vi "Main.vi"() -> ()   [LabVIEW 2023]
uses:
  #type_def_Cafe_Additions.ctl
  #type_def_States.ctl
  #type_def_Coffee_Data.ctl
  #type_def_Timing.ctl
  <vilib>/Utility/file.llb/Write Delimited Spreadsheet (string).vi
panel:
  out "error out":errorcluster
  in  "error in":errorcluster
  in  "Stop":bool
  out "Cafe Additions":T1
  in  "Cafe Mocha":bool
  in  "Cafe Latte":bool
  in  "Espresso Macchiato":bool
  in  "Espresso":bool
  # "WYBIERZ KAWÊ:"
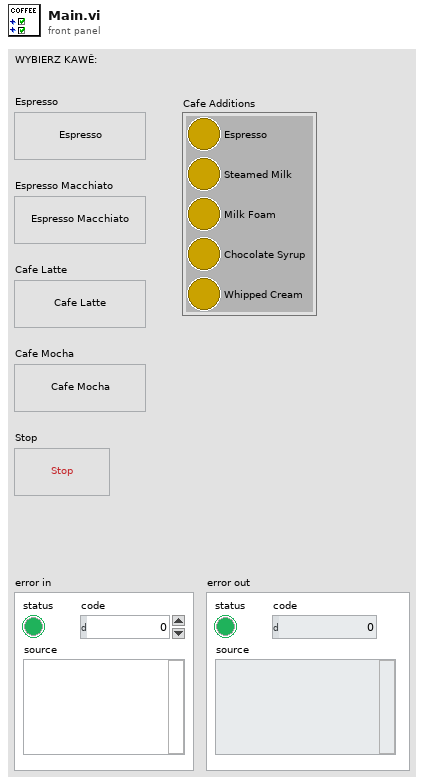
[diagram p1: front panel]
types:
  T1 = typedef "#type_def_Cafe_Additions.ctl" = cluster{"Espresso":bool, "Steamed Milk":bool, "Milk Foam":bool, "Chocolate Syrup":bool, "Whipped Cream":bool}
  T2 = typedef "#type_def_States.ctl" = enum16{"Init", "Idle", "Espresso", "Steamed Milk", "Milk Foam", "Chocolate Syrup", "Whipped Cream", "Stop", "Log"}
  T3 = typedef "#type_def_Coffee_Data.ctl" = cluster{"Cafe Additions":T1, "Timing":T4}
  T4 = typedef "#type_def_Timing.ctl" = cluster{"Espresso":dbl, "Steamed Milk":dbl, "Milk Foam":dbl, "Chocolate Syrup":dbl, "Whipped Cream":dbl}
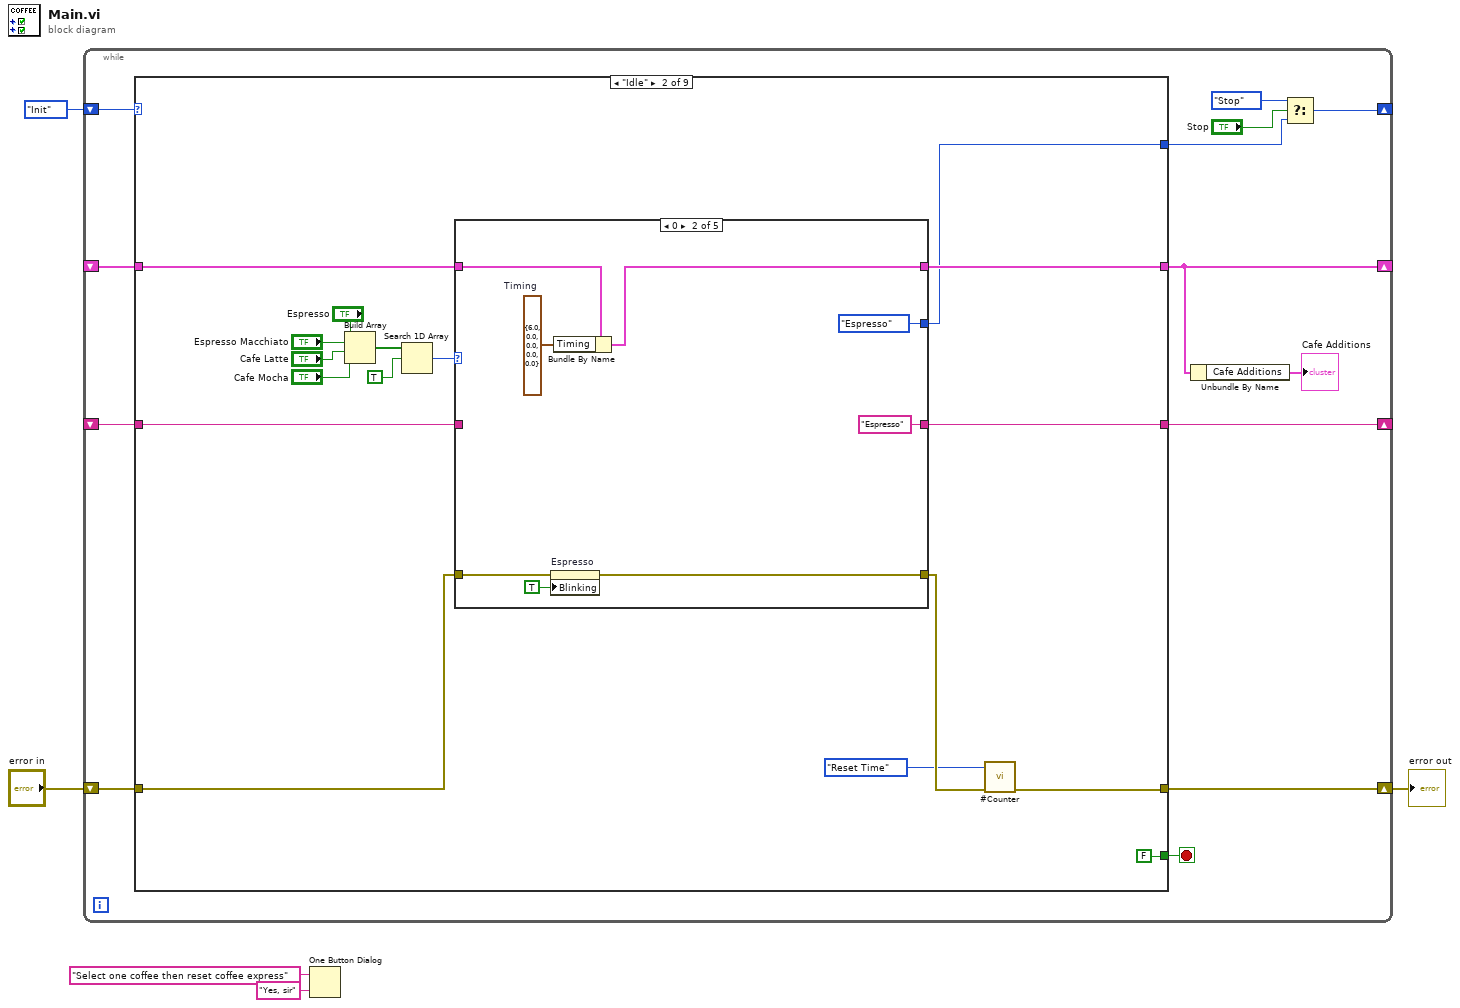
[diagram p0: block diagram]
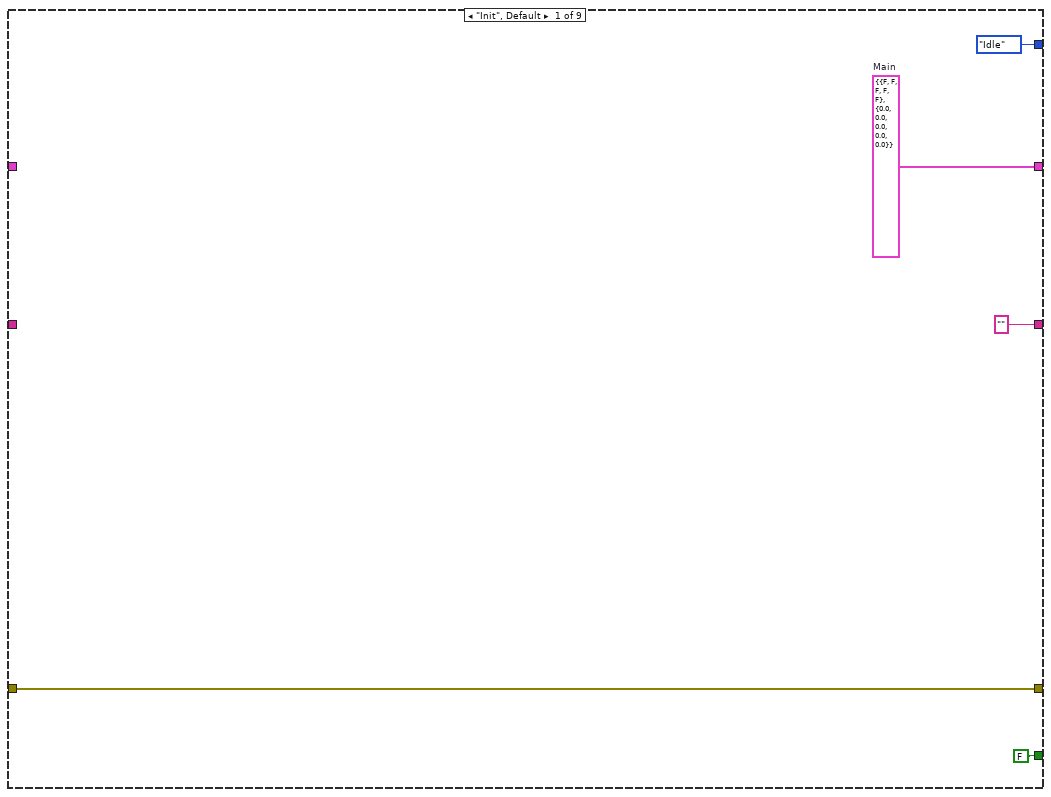
[diagram p2: hidden frame]
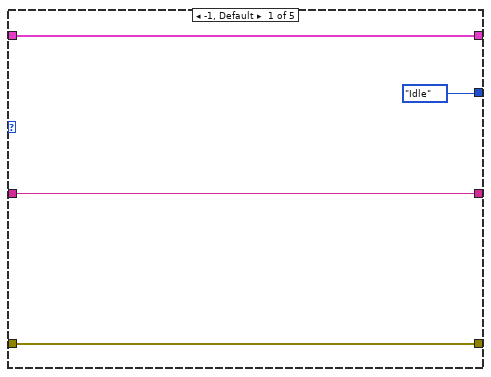
[diagram p3: hidden frame]
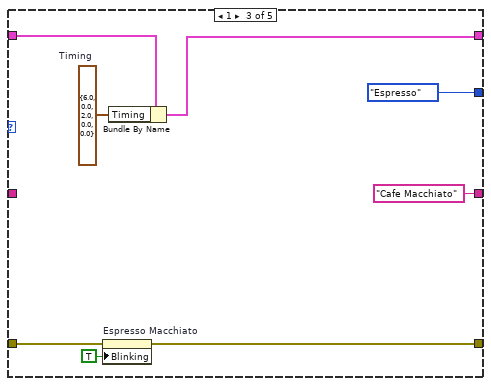
[diagram p4: hidden frame]
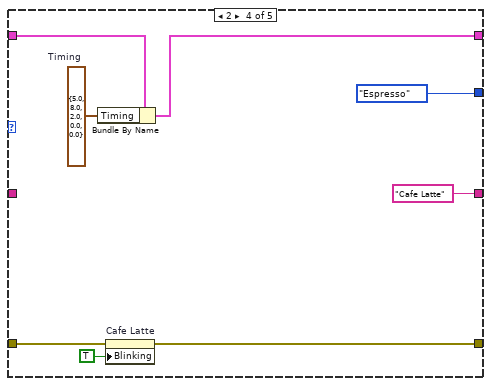
[diagram p5: hidden frame]
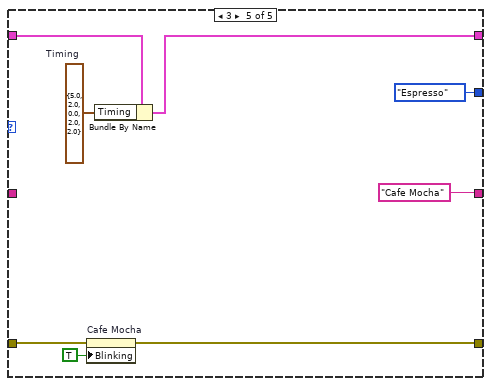
[diagram p6: hidden frame]
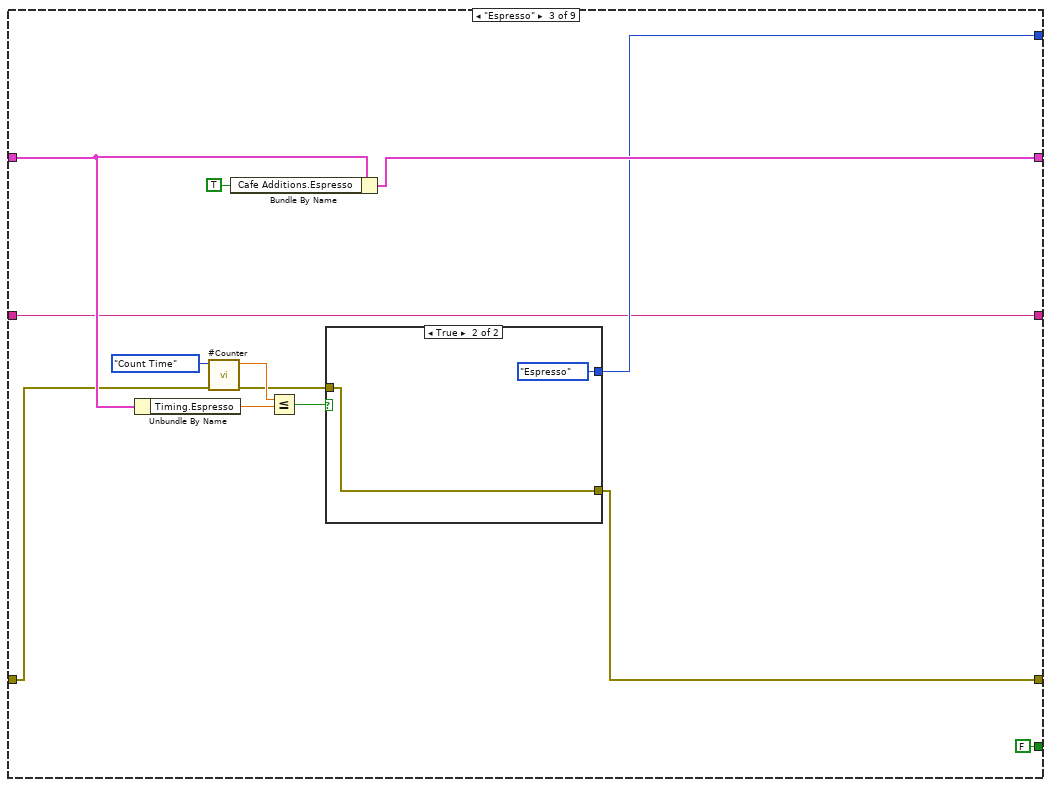
[diagram p7: hidden frame]
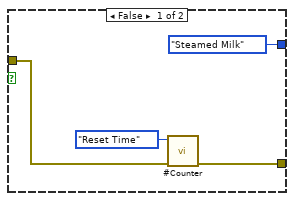
[diagram p8: hidden frame]
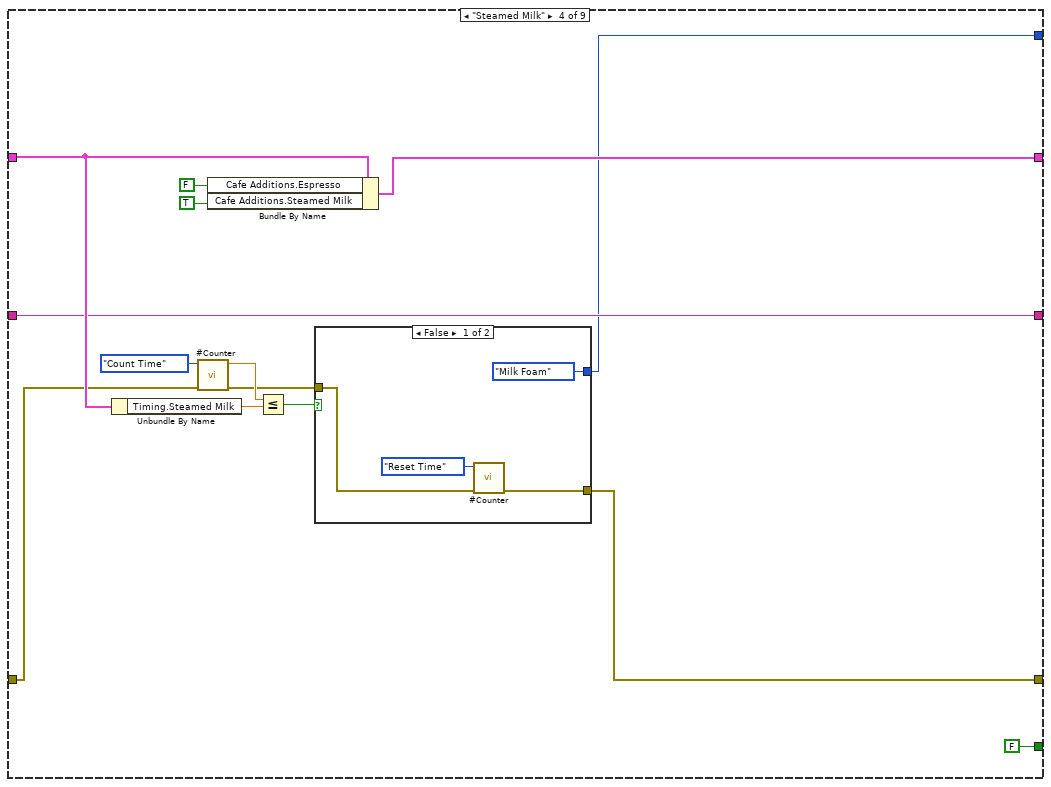
[diagram p9: hidden frame]
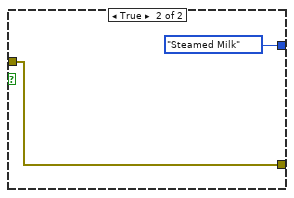
[diagram p10: hidden frame]
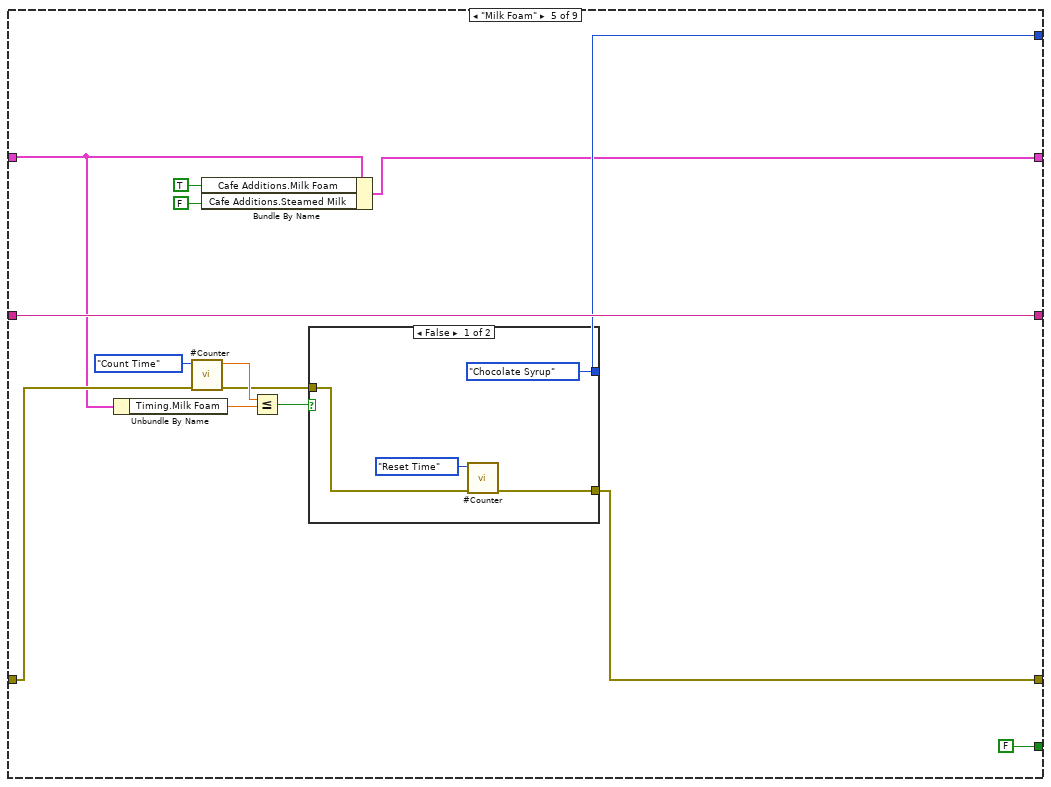
[diagram p11: hidden frame]
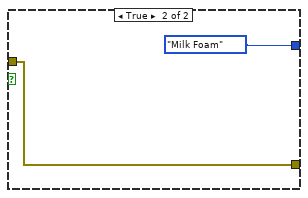
[diagram p12: hidden frame]
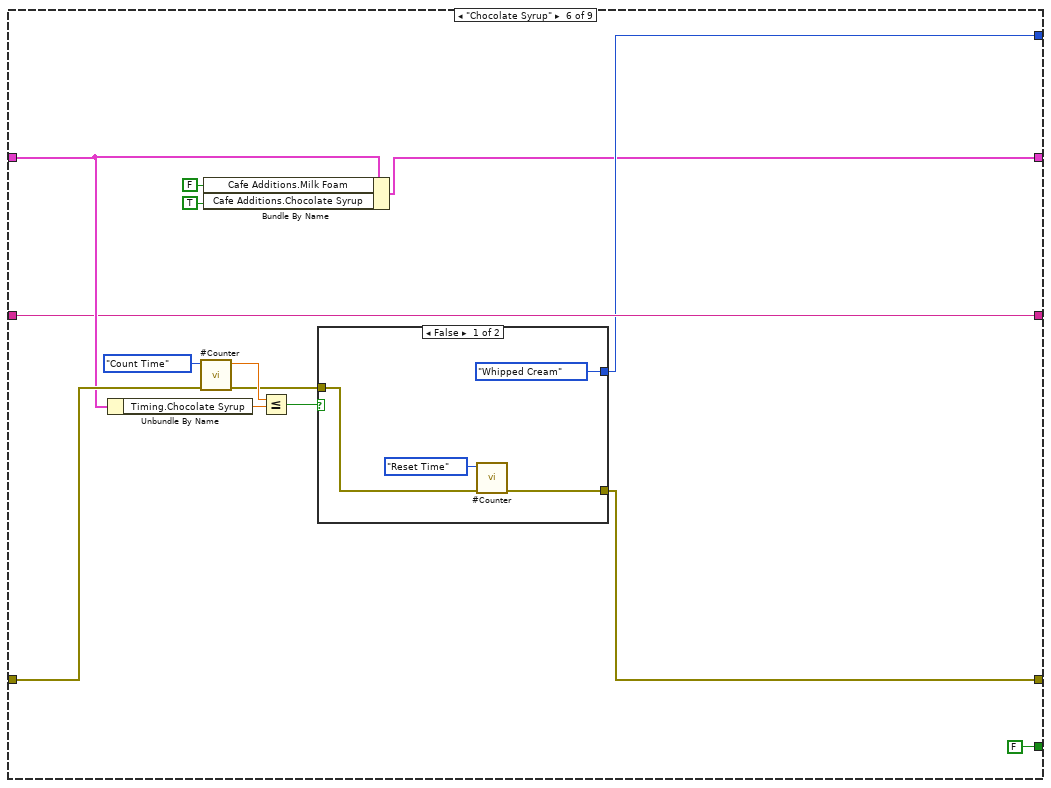
[diagram p13: hidden frame]
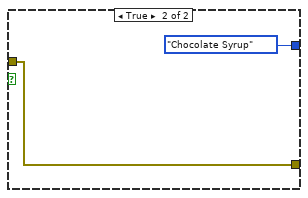
[diagram p14: hidden frame]
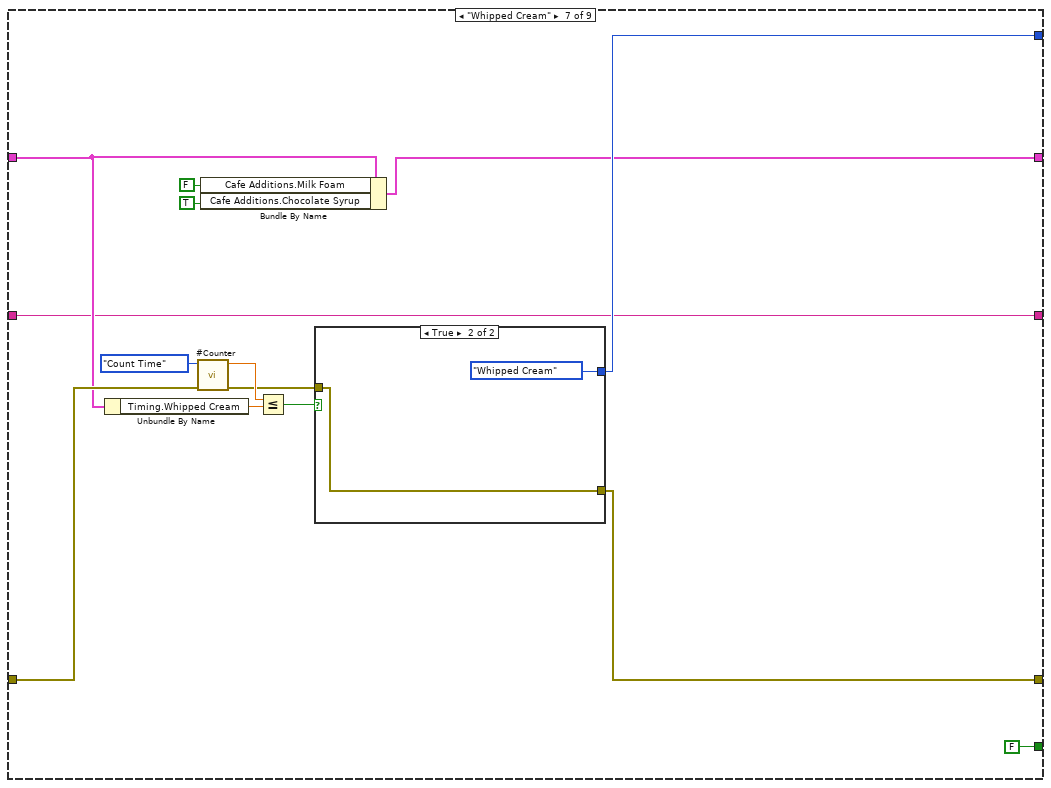
[diagram p15: hidden frame]
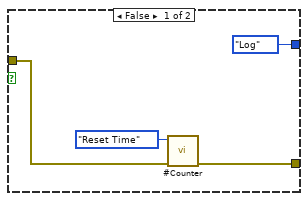
[diagram p16: hidden frame]
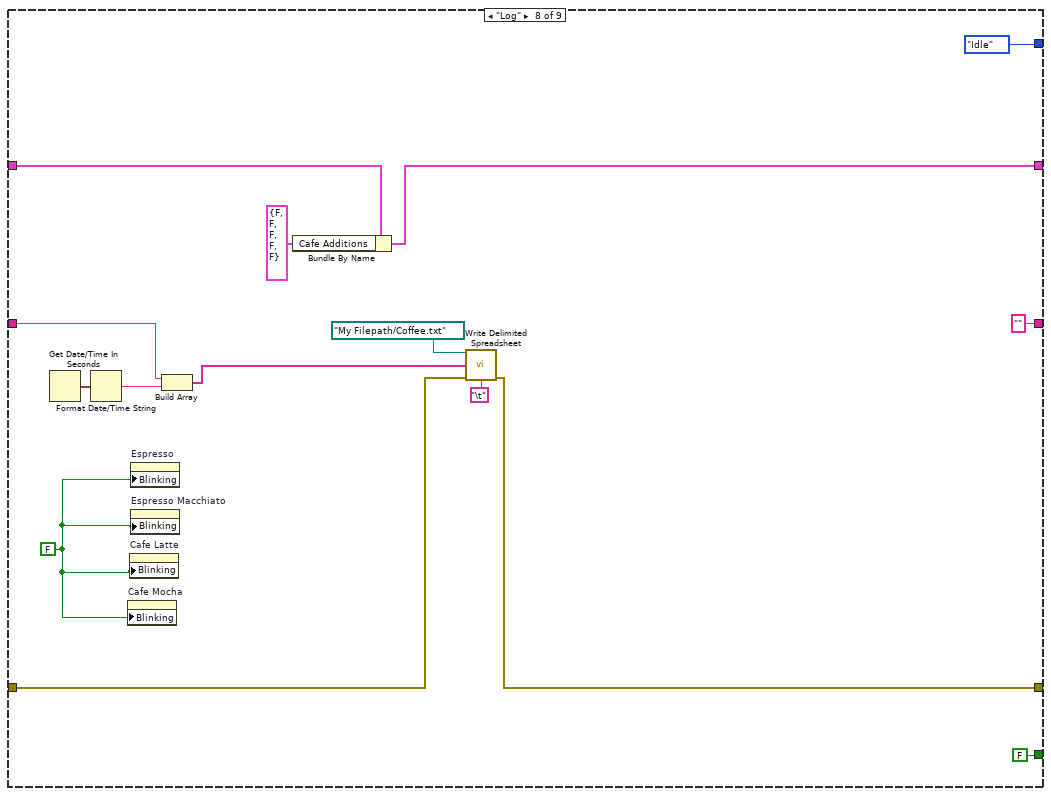
[diagram p17: hidden frame]
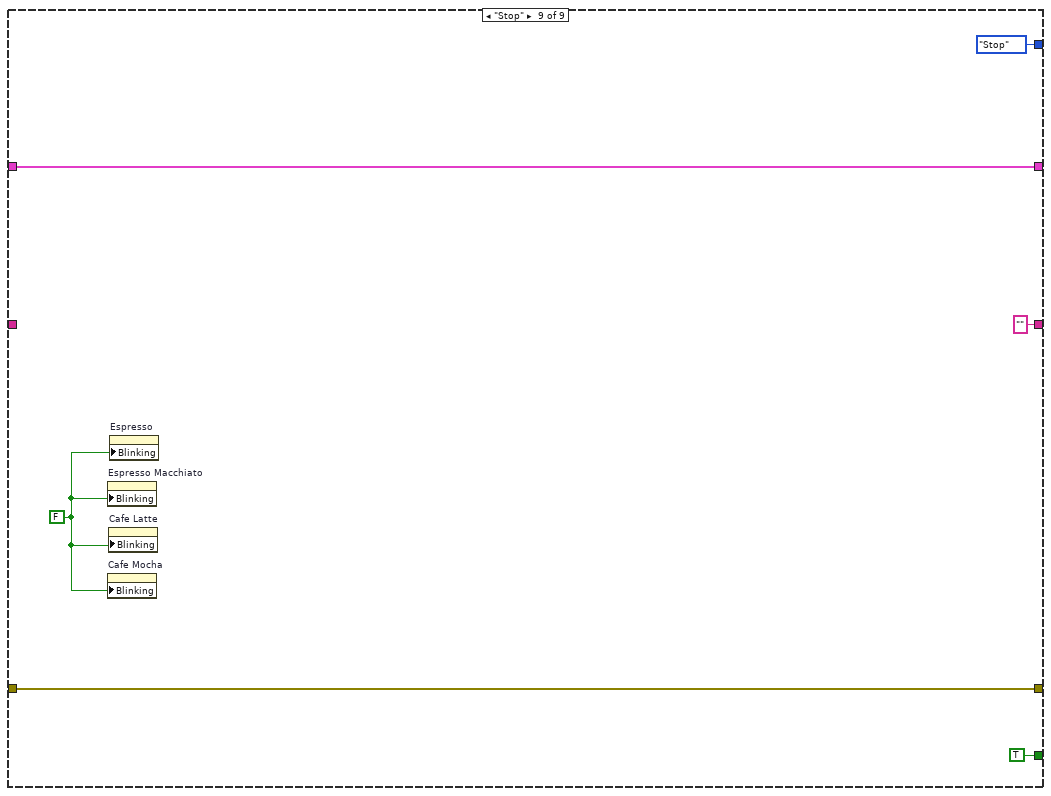
[diagram p18: hidden frame]
diagram:
  n1 = while {
    shift-right: [w17] -> w4
    shift-left: "error in" -> [w18]
    shift-right: [w6] -> _
    shift-left: #type_def_States."Init" -> [w16]
    shift-right: [w15] -> _
    shift-left: _ -> [w12]
    shift-right: [w13] -> _
    shift-left: _ -> [w11]
    stop <- w10 stop-if-true
    n2 = case shown="\"Idle\"" w16 {
      tunnel: w18 -> [w21 w37 w82 w102 w122 w141 w161 w189 w195]
      tunnel: [w21 w26 w80 w97 w119 w136 w159 w188 w195] -> w17
      tunnel: [w23 w33 w88 w100 w116 w137 w157 w183 w194] -> w15
      tunnel: ["" w35 w78 w101 w123 w139 w156 "" ""] -> w13
      tunnel: w12 -> [_ w34 w87 w103 w121 w140 w160 w184 w194]
      tunnel: w11 -> [_ w36 w78 w101 w123 w139 w156 w180 _]
      tunnel: [FALSE FALSE FALSE FALSE FALSE FALSE FALSE FALSE TRUE] -> w10
      tunnel: [#type_def_States."Idle" w32 w84 w96 w117 w138 w158 #type_def_States."Idle" #type_def_States."Stop"] -> w7
      frame "Init", Default {
        w23 = T3 {"Cafe Additions"={"Espresso"=FALSE, "Steamed Milk"=FALSE, "Milk Foam"=FALSE, "Chocolate Syrup"=FALSE, "Whipped Cream"=FALSE}, "Timing"={"Espresso"=0.0, "Steamed Milk"=0.0, "Milk Foam"=0.0, "Chocolate Syrup"=0.0, "Whipped Cream"=0.0}}  # Main
      }
      frame "Idle" {
        n3 = Build Array("Espresso", "Espresso Macchiato", "Cafe Latte", "Cafe Mocha") -> (w40:bool[])
        n4 = Search 1D Array(1D array=w40, element=TRUE) -> (index of element=w38:i32)  [unwired: 1 in]
        n5 = case shown="0" w38 {
          tunnel: w37 -> [w44 w47 w55 w63 w71]
          tunnel: [w44 w46 w54 w62 w70] -> w25
          tunnel: w36 -> [w43 _ _ _ _]
          tunnel: [w43 "Espresso" "Cafe Macchiato" "Cafe Latte" "Cafe Mocha"] -> w35
          tunnel: w34 -> [w42 w50 w59 w67 w73]
          tunnel: [w42 w49 w58 w66 w72] -> w33
          tunnel: [#type_def_States."Idle" #type_def_States."Espresso" #type_def_States."Espresso" #type_def_States."Espresso" #type_def_States."Espresso"] -> w32
          frame -1, Default {
          }
          frame 0 {
            w51 = T4 {"Espresso"=6.0, "Steamed Milk"=0.0, "Milk Foam"=0.0, "Chocolate Syrup"=0.0, "Whipped Cream"=0.0}  # Timing
            n6 = property on="Espresso" class="Bool"(error in=w47, "Blinking"=TRUE) -> (error out=w46:errorcluster)  [unwired: 1 in, 1 out]
            n7 = Bundle By Name(cluster=w50, "Timing"=w51) -> (w49:T3)
          }
          frame 1 {
            w60 = T4 {"Espresso"=6.0, "Steamed Milk"=0.0, "Milk Foam"=2.0, "Chocolate Syrup"=0.0, "Whipped Cream"=0.0}  # Timing
            n8 = property on="Espresso Macchiato" class="Bool"(error in=w55, "Blinking"=TRUE) -> (error out=w54:errorcluster)  [unwired: 1 in, 1 out]
            n9 = Bundle By Name(cluster=w59, "Timing"=w60) -> (w58:T3)
          }
          frame 2 {
            w68 = T4 {"Espresso"=5.0, "Steamed Milk"=8.0, "Milk Foam"=2.0, "Chocolate Syrup"=0.0, "Whipped Cream"=0.0}  # Timing
            n10 = Bundle By Name(cluster=w67, "Timing"=w68) -> (w66:T3)
            n11 = property on="Cafe Latte" class="Bool"(error in=w63, "Blinking"=TRUE) -> (error out=w62:errorcluster)  [unwired: 1 in, 1 out]
          }
          frame 3 {
            w76 = T4 {"Espresso"=5.0, "Steamed Milk"=2.0, "Milk Foam"=0.0, "Chocolate Syrup"=2.0, "Whipped Cream"=2.0}  # Timing
            n12 = property on="Cafe Mocha" class="Bool"(error in=w71, "Blinking"=TRUE) -> (error out=w70:errorcluster)  [unwired: 1 in, 1 out]
            n13 = Bundle By Name(cluster=w73, "Timing"=w76) -> (w72:T3)
          }
        }
        n14 = call "#Counter.vi"("error in"=w25, "Enum"=enum16{"Count Time", "Pause Time", "Reset Time"}."Reset Time") -> ("error out"=w26:errorcluster)  [unwired: 8 in, 1 out]
      }
      frame "Espresso" {
        n15 = Unbundle By Name(w87) -> ("Timing.Espresso"=w86:dbl)
        n16 = call "#Counter.vi"("error in"=w82, "Enum"=enum16{"Count Time", "Pause Time", "Reset Time"}."Count Time") -> ("error out"=w81:errorcluster, "Elapsed Time"=w83:dbl)  [unwired: 8 in]
        n17 = Bundle By Name(cluster=w87, "Cafe Additions.Espresso"=TRUE) -> (w88:T3)
        n18 = Less Or Equal?(x=w83, y=w86) -> (x <= y?=w85:bool)
        n19 = case shown="True" w85 {
          tunnel: [#type_def_States."Steamed Milk" #type_def_States."Espresso"] -> w84
          tunnel: w81 -> [w92 w94]
          tunnel: [w91 w94] -> w80
          frame False {
            n20 = call "#Counter.vi"("error in"=w92, "Enum"=enum16{"Count Time", "Pause Time", "Reset Time"}."Reset Time") -> ("error out"=w91:errorcluster)  [unwired: 8 in, 1 out]
          }
          frame True {
          }
        }
      }
      frame "Steamed Milk" {
        n21 = Unbundle By Name(w103) -> ("Timing.Steamed Milk"=w108:dbl)
        n22 = call "#Counter.vi"("error in"=w102, "Enum"=enum16{"Count Time", "Pause Time", "Reset Time"}."Count Time") -> ("error out"=w105:errorcluster, "Elapsed Time"=w106:dbl)  [unwired: 8 in]
        n23 = Bundle By Name(cluster=w103, "Cafe Additions.Espresso"=FALSE, "Cafe Additions.Steamed Milk"=TRUE ("Cafe Additions.Espresso")) -> (w100:T3)
        n24 = Less Or Equal?(x=w106, y=w108) -> (x <= y?=w107:bool)
        n25 = case shown="False" w107 {
          tunnel: [#type_def_States."Milk Foam" #type_def_States."Steamed Milk"] -> w96
          tunnel: w105 -> [w112 w114]
          tunnel: [w111 w114] -> w97
          frame False {
            n26 = call "#Counter.vi"("error in"=w112, "Enum"=enum16{"Count Time", "Pause Time", "Reset Time"}."Reset Time") -> ("error out"=w111:errorcluster)  [unwired: 8 in, 1 out]
          }
          frame True {
          }
        }
      }
      frame "Milk Foam" {
        n27 = Unbundle By Name(w121) -> ("Timing.Milk Foam"=w120:dbl)
        n28 = call "#Counter.vi"("error in"=w122, "Enum"=enum16{"Count Time", "Pause Time", "Reset Time"}."Count Time") -> ("error out"=w126:errorcluster, "Elapsed Time"=w127:dbl)  [unwired: 8 in]
        n29 = Bundle By Name(cluster=w121, "Cafe Additions.Milk Foam"=TRUE ("Cafe Additions.Espresso"), "Cafe Additions.Steamed Milk"=FALSE ("Cafe Additions.Espresso")) -> (w116:T3)
        n30 = Less Or Equal?(x=w127, y=w120) -> (x <= y?=w128:bool)
        n31 = case shown="False" w128 {
          tunnel: [#type_def_States."Chocolate Syrup" #type_def_States."Milk Foam"] -> w117
          tunnel: w126 -> [w132 w134]
          tunnel: [w131 w134] -> w119
          frame False {
            n32 = call "#Counter.vi"("error in"=w132, "Enum"=enum16{"Count Time", "Pause Time", "Reset Time"}."Reset Time") -> ("error out"=w131:errorcluster)  [unwired: 8 in, 1 out]
          }
          frame True {
          }
        }
      }
      frame "Chocolate Syrup" {
        n33 = Unbundle By Name(w140) -> ("Timing.Chocolate Syrup"=w143:dbl)
        n34 = call "#Counter.vi"("error in"=w141, "Enum"=enum16{"Count Time", "Pause Time", "Reset Time"}."Count Time") -> ("error out"=w146:errorcluster, "Elapsed Time"=w147:dbl)  [unwired: 8 in]
        n35 = Bundle By Name(cluster=w140, "Cafe Additions.Milk Foam"=FALSE ("Cafe Additions.Espresso"), "Cafe Additions.Chocolate Syrup"=TRUE ("Cafe Additions.Espresso")) -> (w137:T3)
        n36 = Less Or Equal?(x=w147, y=w143) -> (x <= y?=w148:bool)
        n37 = case shown="False" w148 {
          tunnel: [#type_def_States."Whipped Cream" #type_def_States."Chocolate Syrup"] -> w138
          tunnel: w146 -> [w152 w154]
          tunnel: [w151 w154] -> w136
          frame False {
            n38 = call "#Counter.vi"("error in"=w152, "Enum"=enum16{"Count Time", "Pause Time", "Reset Time"}."Reset Time") -> ("error out"=w151:errorcluster)  [unwired: 8 in, 1 out]
          }
          frame True {
          }
        }
      }
      frame "Whipped Cream" {
        n39 = Unbundle By Name(w160) -> ("Timing.Whipped Cream"=w163:dbl)
        n40 = call "#Counter.vi"("error in"=w161, "Enum"=enum16{"Count Time", "Pause Time", "Reset Time"}."Count Time") -> ("error out"=w166:errorcluster, "Elapsed Time"=w167:dbl)  [unwired: 8 in]
        n41 = Bundle By Name(cluster=w160, "Cafe Additions.Milk Foam"=FALSE ("Cafe Additions.Espresso"), "Cafe Additions.Chocolate Syrup"=TRUE ("Cafe Additions.Espresso")) -> (w157:T3)
        n42 = Less Or Equal?(x=w167, y=w163) -> (x <= y?=w168:bool)
        n43 = case shown="True" w168 {
          tunnel: [#type_def_States."Log" #type_def_States."Whipped Cream"] -> w158
          tunnel: w166 -> [w172 w174]
          tunnel: [w171 w174] -> w159
          frame False {
            n44 = call "#Counter.vi"("error in"=w172, "Enum"=enum16{"Count Time", "Pause Time", "Reset Time"}."Reset Time") -> ("error out"=w171:errorcluster)  [unwired: 8 in, 1 out]
          }
          frame True {
          }
        }
      }
      frame "Log" {
        w190 = FALSE
        n45 = Get Date/Time In Seconds() -> (seconds since 1Jan1904=w182:timestamp)
        n46 = Format Date/Time String(seconds (now)=w182) -> (date/time string=w181:string)  [unwired: 2 in]
        n47 = property on="Cafe Mocha" class="Bool"("Blinking"=w190) -> ()  [unwired: 2 in, 2 out]
        n48 = property on="Cafe Latte" class="Bool"("Blinking"=w190) -> ()  [unwired: 2 in, 2 out]
        n49 = property on="Espresso" class="Bool"("Blinking"=w190) -> ()  [unwired: 2 in, 2 out]
        n50 = property on="Espresso Macchiato" class="Bool"("Blinking"=w190) -> ()  [unwired: 2 in, 2 out]
        n51 = Build Array(w180, w181) -> (w179:string[])
        n52 = Bundle By Name(cluster=w184, "Cafe Additions"=T1 {"Espresso"=FALSE, "Steamed Milk"=FALSE, "Milk Foam"=FALSE, "Chocolate Syrup"=FALSE, "Whipped Cream"=FALSE}) -> (w183:T3)
        n53 = call-poly <vilib>:"Write Delimited Spreadsheet.vi"("file path (dialog if empty)"=path "My Filepath/Coffee.txt", "1D data"=w179, "error in (no error)"=w189, "delimiter (\\t)"="\t") -> ("error out"=w188:errorcluster)  [unwired: 10 in, 1 out]
      }
      frame "Stop" {
        w191 = FALSE
        n54 = property on="Espresso Macchiato" class="Bool"("Blinking"=w191) -> ()  [unwired: 2 in, 2 out]
        n55 = property on="Cafe Mocha" class="Bool"("Blinking"=w191) -> ()  [unwired: 2 in, 2 out]
        n56 = property on="Cafe Latte" class="Bool"("Blinking"=w191) -> ()  [unwired: 2 in, 2 out]
        n57 = property on="Espresso" class="Bool"("Blinking"=w191) -> ()  [unwired: 2 in, 2 out]
      }
    }
    n58 = Unbundle By Name(w15) -> ("Cafe Additions"=→"Cafe Additions":T1)
    n59 = Select(t=#type_def_States."Stop", s="Stop", f=w7) -> (s? t:f=w6:T2)
  }
  "error out" <- w4
  n60 = One Button Dialog(message="Select one coffee then reset coffee express", button name ("OK")="Yes, sir") -> ()  [unwired: 1 out]
